vi "finish5RobotsNormalGamePlay.vi"(8 "error in (no error)":errorcluster, 10 "Game":refnum<class "Game.lvclass">, 11 "5RobotsNormalGamePlay in":refnum<class "5RobotsNormalGamePlay.lvclass">) -> (0 "error out":errorcluster, 1 "Game out":refnum<class "Game.lvclass">, 2 "finish?":bool, 3 "5RobotsNormalGamePlay out":refnum<class "5RobotsNormalGamePlay.lvclass">)   [LabVIEW 2023, in "5RobotsNormalGamePlay.lvclass"]
uses:
  5RobotsNormalGamePlay.lvclass
  C:/Users/ebert/Desktop/roboime/SSL_AI/Play_class/Play.lvclass
  Game_class/Game.lvclass
  Play_class/Play.lvclass
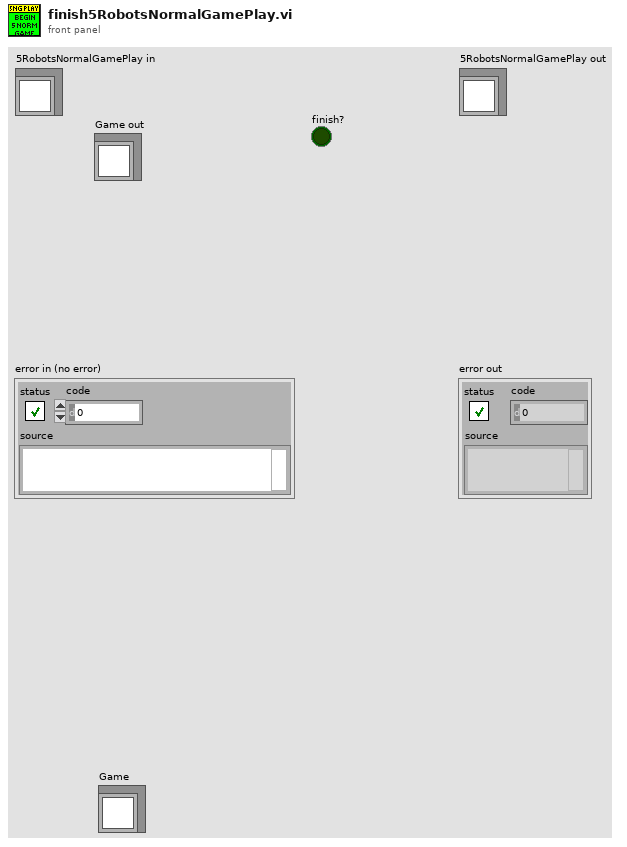
[diagram p1: front panel]
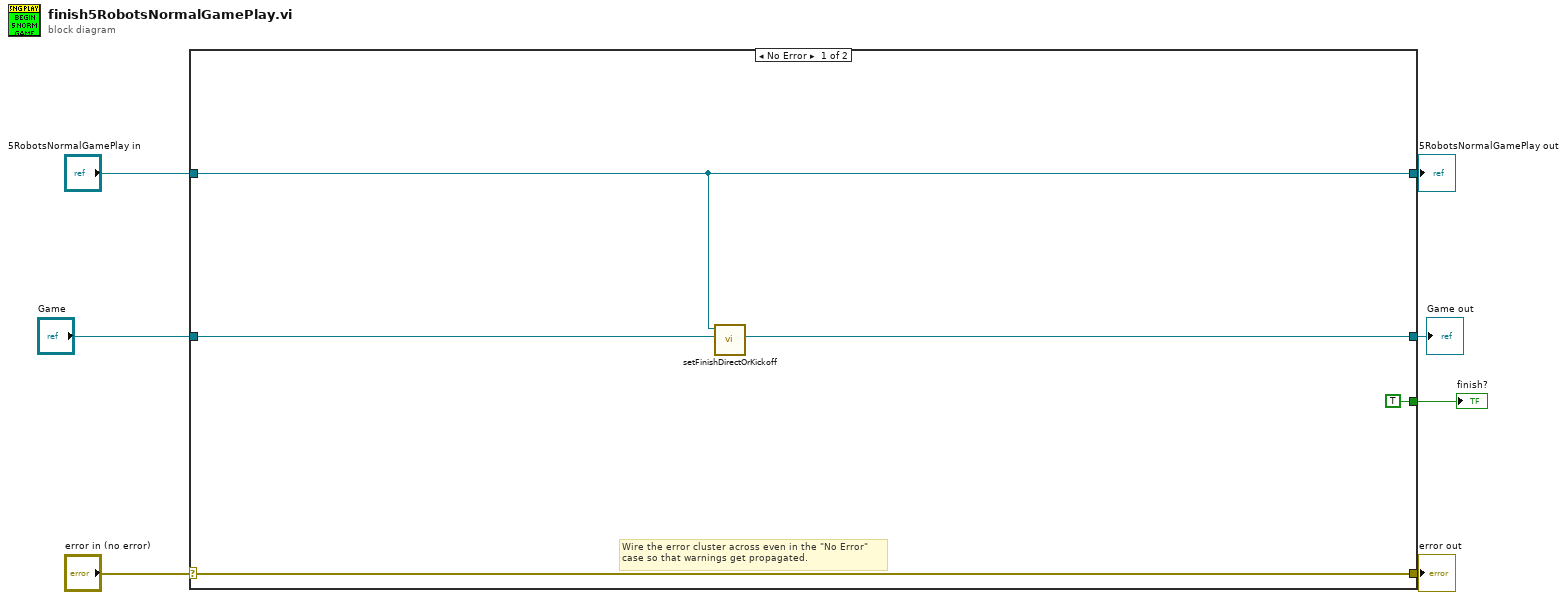
[diagram p0: block diagram]
diagram:
  n1 = case shown="No Error" "error in (no error)" {
    selector: "error in (no error)" -> [w12 w14]
    tunnel: [w12 w14] -> w6
    tunnel: [w10 w13] -> w4
    tunnel: "5RobotsNormalGamePlay in" -> [w10 w13]
    tunnel: [TRUE _] -> w3
    tunnel: "Game" -> [w9 _]
    tunnel: [w8 _] -> w1
    frame No Error {
      # "Wire the error cluster across even in the \"No Error\"\ncase so that warnings get propagated."
      n2 = call "setFinishDirectOrKickoff.vi"("Game"=w9, "Play in"=w10) -> ("Game out"=w8:refnum<class "Game.lvclass">)  [unwired: 7 in, 2 out]
    }
    frame Error {
    }
  }
  "error out" <- w6
  "5RobotsNormalGamePlay out" <- w4
  "finish?" <- w3
  "Game out" <- w1
